vi "CALC_PAR_CAT.vi"(0 "VISA IN":refnum<visa-resource-name>, 5 "error in":errorcluster, 7 "Channel":i32=1) -> (11 "Type":string, 13 "Meas":string, 14 "VISA Out":refnum<visa-resource-name>, 16 "Data":string, 19 "error out":errorcluster)   [LabVIEW 2018, in "PNA-X.lvlib"]
doc: "CALCulate<cnum>:PARameter:CATalog? \n(Read-only) Returns the names and parameters of existing measurements for the specified channel. \nNote: For Balanced Measurements: CALC:PAR:CAT? may have an unexpected behavior. Learn \nmore. \nSee Critical Note \nParameters \n<cnum> Channel number of the measurements to be listed. If unspecified, <cnum> is \nset to 1. \nExamples CALC:PAR:CAT? \ncalculate2:parameter:catalog? \nReturn Type String - \"<measurement name>,<parameter>,[<measurement \nname>,<parameter>...]\" \n1553\n\nDefault \"CH1_S11_1,S11\""
uses:
  PNA-X.lvlib
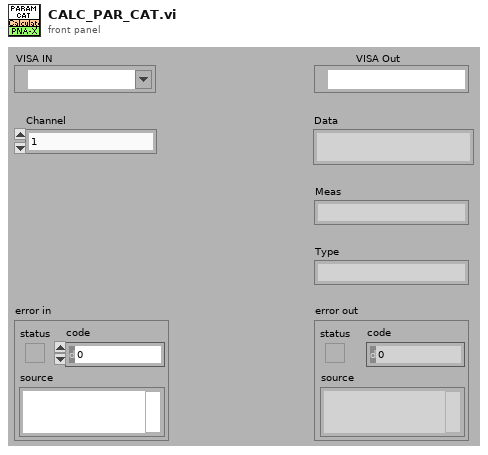
[diagram p1: front panel]
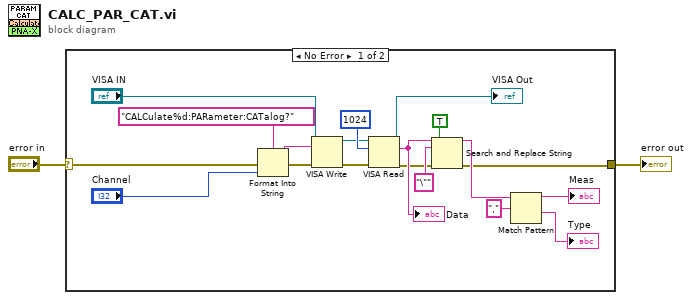
[diagram p0: block diagram]
diagram:
  n1 = case shown="No Error" "error in" {
    selector: "error in" -> [w21 w22]
    tunnel: [w3 w22] -> w1
    frame No Error {
      n2 = Format Into String(format string="CALCulate%d:PARameter:CATalog?" ("Cmdline"), error in=w21, "Channel") -> (resulting string=w19:string, error out=w20:errorcluster)  [unwired: 1 in]
      n3 = VISA Write(VISA resource name="VISA IN", write buffer=w19, error in (no error)=w20) -> (VISA resource name out=w14:refnum<visa-resource-name>, error out=w16:errorcluster)  [unwired: 1 out]
      n4 = VISA Read(VISA resource name=w14, byte count=1024, error in (no error)=w16) -> (VISA resource name out=→"VISA Out":refnum<visa-resource-name>, read buffer=w8:string, error out=w4:errorcluster)  [unwired: 1 out]
      "Data" <- w8
      n5 = Search and Replace String(replace all?=TRUE ("replace all? (F)"), input string=w8, search string="\"", error in=w4) -> (result string=w5:string, error out=w3:errorcluster)  [unwired: 4 in, 2 out]
      n6 = Match Pattern(string=w5, regular expression=",") -> (before substring=→"Meas":string, after substring=→"Type":string)  [unwired: 1 in, 2 out]
    }
    frame Error {
    }
  }
  "error out" <- w1
